vi "List Roots.vi"(10 "Optional Root Name":string, 11 "Tree Map In":T1) -> (1 "Ordered Unique Root Paths":string[](array[string]), 3 "Unique Root Paths Set":set{string}(c389))   [LabVIEW 2020, in "Tree Map.lvlib"]
doc: "Iterates through all tree nodes and finds the root nodes. This feature is designed only for the Tree Map, since an XML document cannot contain more than 1 root.\n\n<b>Author:</b> Piotr Kruczkowski <PrimaryKey>\n<b>License:</b> NewBSD\n\nCopyright (c) 2019, National Instruments\nAll rights reserved.\n\nRedistribution and use in source and binary forms, with or without\nmodification, are permitted provided that the following conditions are met:\n1. Redistributions of source code must retain the above copyright\n notice, this list of conditions and the following disclaimer.\n2. Redistributions in binary form must reproduce the above copyright\n notice, this list of conditions and the following disclaimer in the\n documentation and/or other materials provided with the distribution.\n3. Neither the name of National Instruments nor the\n names of its contributors may be used to endorse or promote products\n derived from this software without specific prior written permission.\n\nTHIS SOFTWARE IS PROVIDED BY National Instruments ''AS IS'' AND ANY\nEXPRESS OR IMPLIED WARRANTIES, INCLUDING, BUT NOT LIMITED TO, THE IMPLIED\nWARRANTIES OF MERCHANTABILITY AND FITNESS FOR A PARTICULAR PURPOSE ARE\nDISCLAIMED. IN NO EVENT SHALL National Instruments BE LIABLE FOR ANY\nDIRECT, INDIRECT, INCIDENTAL, SPECIAL, EXEMPLARY, OR CONSEQUENTIAL DAMAGES\n(INCLUDING, BUT NOT LIMITED TO, PROCUREMENT OF SUBSTITUTE GOODS OR SERVICES;\nLOSS OF USE, DATA, OR PROFITS; OR BUSINESS INTERRUPTION) HOWEVER CAUSED AND\nON ANY THEORY OF LIABILITY, WHETHER IN CONTRACT, STRICT LIABILITY, OR TORT\n(INCLUDING NEGLIGENCE OR OTHERWISE) ARISING IN ANY WAY OUT OF THE USE OF THIS\nSOFTWARE, EVEN IF ADVISED OF THE POSSIBILITY OF SUCH DAMAGE."
uses:
  Tree Map.lvlib
  Tree Map Data.ctl
  Utility/Join Strings Tree.vi
  SubVIs/TM Head and Tail.vi
  SubVIs/TM Init and Last.vi
  Utility/Split String Tree.vi
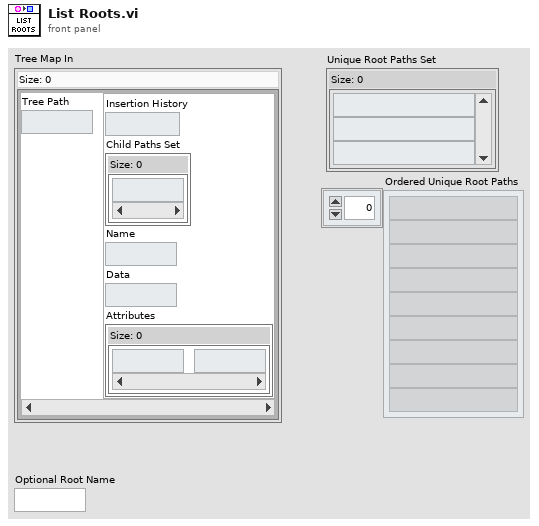
[diagram p1: front panel]
types:
  T1 = typedef "Tree Map.lvlib/Tree Map Data.ctl" = map{string, cluster{"Insertion History":i32, "Child Paths Set":set{string}, "Name":string, "Data":string, "Attributes":map{string, string}}}
  T2 = cluster{"Insertion History":i32, "Tree Path":string}
  T3 = cluster{"Insertion History":i32, "Tree Path":string}[]
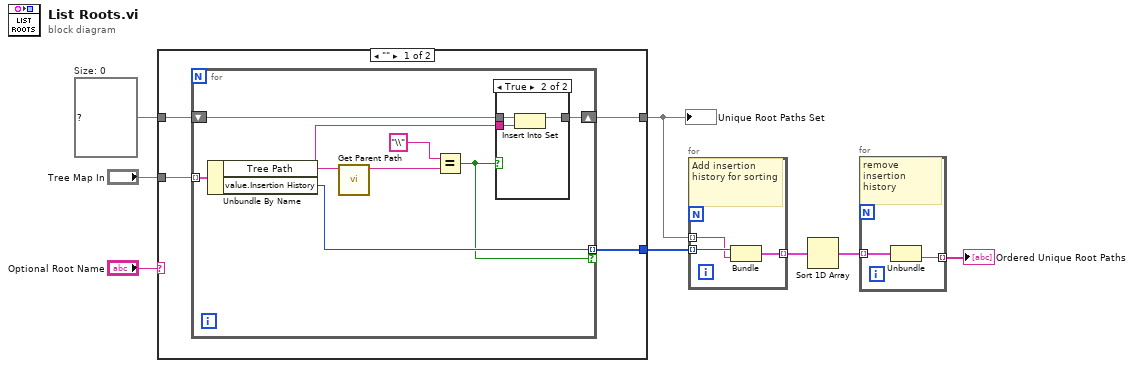
[diagram p0: block diagram]
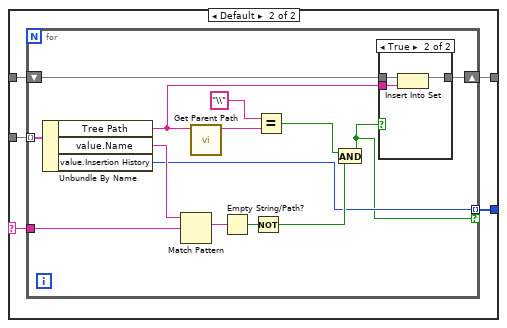
[diagram p3: hidden frame]
diagram:
  w7 = set{string} {}  # Size: 0
  n1 = case shown="\"\"" "Optional Root Name" {
    selector: "Optional Root Name" -> [_ w26]
    tunnel: "Tree Map In" -> [w10 w29]
    tunnel: w7 -> [w12 w28]
    tunnel: [w11 w27] -> w5
    tunnel: [w9 w25] -> w4
    frame "" {
      n2 = for {
        tunnel: w10 -> [w20] mode=indexing
        shift-right: [w18] -> w11
        shift-left: w12 -> [w17]
        tunnel: [w14] -> w9 mode=indexing if=w13
        n3 = Unbundle By Name(w20) -> ("Tree Path"=w19:string, "value.Insertion History"=w14:i32)
        n4 = call "Get Parent Path.vi"("Node Path"=w19) -> ("Parent Path"=w15:string)  [unwired: 8 in, 2 out]
        n5 = Equal?(x="\\", y=w15) -> (x = y?=w13:bool)
        n6 = case shown="True" w13 {
          tunnel: w19 -> [_ w24]
          tunnel: [w21 w23] -> w18
          tunnel: w17 -> [w21 w22]
          frame False {
          }
          frame True {
            n7 = Insert Into Set(10:w24, 11:w22) -> (3:w23:set{string})  [unwired: 1 out]
          }
        }
      }
    }
    frame Default {
      n8 = for {
        tunnel: w29 -> [w43] mode=indexing
        shift-right: [w41] -> w27
        shift-left: w28 -> [w40]
        tunnel: w26 -> [w38]
        tunnel: [w31] -> w25 mode=indexing if=w30
        n9 = Unbundle By Name(w43) -> ("Tree Path"=w42:string, "value.Name"=w37:string, "value.Insertion History"=w31:i32)
        n10 = Match Pattern(string=w37, regular expression=w38) -> (match substring=w39:string)  [unwired: 1 in, 3 out]
        n11 = call "Get Parent Path.vi"("Node Path"=w42) -> ("Parent Path"=w34:string)  [unwired: 8 in, 2 out]
        n12 = Empty String/Path?(string/path=w39) -> (empty?=w36:bool)
        n13 = Not(x=w36) -> (.not. x?=w35:bool)
        n14 = Equal?(x="\\", y=w34) -> (x = y?=w32:bool)
        n15 = And(x=w32, y=w35) -> (x .and. y?=w30:bool)
        n16 = case shown="True" w30 {
          tunnel: w42 -> [_ w47]
          tunnel: [w44 w46] -> w41
          tunnel: w40 -> [w44 w45]
          frame False {
          }
          frame True {
            n17 = Insert Into Set(10:w47, 11:w45) -> (3:w46:set{string})  [unwired: 1 out]
          }
        }
      }
    }
  }
  "Unique Root Paths Set" <- w5
  n18 = for {
    tunnel: w5 -> [w49] mode=indexing
    tunnel: w4 -> [w50] mode=indexing
    tunnel: [w48] -> w3 mode=indexing
    # "Add insertion history for sorting"
    n19 = Bundle("Insertion History"=w50, "Tree Path"=w49) -> (w48:T2)  [unwired: 1 in]
  }
  n20 = Sort 1D Array(array=w3) -> (sorted array=w2:T3)
  n21 = for {
    tunnel: w2 -> [w52] mode=indexing
    tunnel: [w51] -> w1 mode=indexing
    # "remove insertion history"
    n22 = Unbundle(w52) -> ("Tree Path"=w51:string)  [unwired: 1 out]
  }
  "Ordered Unique Root Paths" <- w1
